vi "FDD Self TRAINING Parse Datafile Into BINS Ver05.vi"(9 "Zone Density \n(KEEP Closest # Points)":i32=5, 10 "Data BINS Defined - ARRAY":T2(array[cluster])=[{"Datafile COL"=182.0, "Start Center Value"=60.0, "Bin Width"=5.0, "End Center Value"=100.0}, {"Datafile COL"=83.0, "Start Center Value"=40.0, "Bin Width"=5.0, "End Center Value"=100.0}, {"Datafile COL"=195.0, "Start Center Value"=60.0, "Bin Width"=5.0, "End Center Value"=120.0}], 11 "Input Datafile":path=path "C:/Vance/FDD Split System Project/FDD_LOW-HIGH_EfficiencyHP_Testing/Goodman 14SEER/SHORT LINESET DATA/COOLING/NF - No Fault Cooling Test DATA/NF-SHORT-COOL-SSData 170719a.txt") -> (3 "BEST (Closest in Datafile) Array - String with BIN ASSIGNMENTS":string[][](array[string]), 4 "Each BIN Best Points Array - STRING":string[][](array[string]), 5 "ALL BINS as DEFINED by Start, Width and End, Array - Numeric":dbl[][](array[numeric]))   [LabVIEW 2017]
uses:
  <vilib>/Analysis/Matrix/Datatypes/RealMatrix.ctl
  <vilib>/Utility/file.llb/Read Delimited Spreadsheet (string).vi
  <vilib>/Analysis/Matrix/Numeric/Conversions/Array To Matrix - RA.vi
  <vilib>/Analysis/Matrix/Numeric/Conversions/Matrix To Array - RM.vi
  <vilib>/Utility/file.llb/Write Delimited Spreadsheet (string).vi
  <vilib>/Analysis/Matrix/NI_Matrix.lvlib
  <vilib>/Analysis/NI_AALBase.lvlib
panel:
  out "Total # POINTS":i32
  out "Total # of BINS":i32
  out "Total # POINTS\nKEPT out of\nCurrent Datafile":i32
  out "# RAW Data ROWS":i32
  out "Dmax":dbl format="%.3f"
  out "% Retained":dbl format="%#.2f"
  out "TIME to PARSE (sec)":dbl format="%.2f"
  out "Processing":string
  out "Current Datafile":string
  out "Running":bool
  in  "Tab Control":T1(tab)
  in  "Delete Bins Where\nIndependent Variable #1 > #0":bool=TRUE
  out "Datafile Array - String":string[][](array[string])
  in  "Delete Bins Where\nIndependent Variable #2 > #1":bool
  in  "Delete Bins Where\nIndependent Variable #2 < #0":bool=TRUE
  out "Each Point in Just ONE BIN\n(Distance, BIN#, POINT#)":dbl[][](array[numeric])
  out "BIN RANGES as DEFINED by Start, Width and End Array - Numeric":dbl[][](array[numeric])
  out "RAW Data COLS Selected to be Put into BINS Array - String":string[][](array[string])
  out "Raw Independent Variables STATISTICS - Array":T3(array[cluster])
  out "EACH BIN \nHas X Best\nPOINTS":i32
  out "ALL BINS (Distance, BIN#, POINT#)":dbl[][](array[numeric])
  out "FILTERED by DMAX with Same Point in Multiple BINS Possibly\nDISTANCE, BIN#, POINT# (DATA ARRAY INDEX)":dbl[][](array[numeric])
  out "RAW Data COLS Selected to be Put into BINS Array - String 2":string[][](array[string])
  out "BINNED Data STATISTICS - Array":T3(array[cluster])
  out "PDF Filename":string
  in  "Create PDF Report":bool
  in  "SAVE File":bool
  in  "SAVED Data BINS File Path Control":path
  out "SAVE FILE error out":errorcluster
  out "CREATE JPG error out":errorcluster
  # "Define the BINS.  BIN has a Start Center Value, End Center Value, and Bin Width."
  # "This allows me to delete BINS where\nthe indoor dewpoint is greater than the dry-bulb, or \nwhere outdoor dry-bulb is less than indoor dry-bulb."
  # "POINT# corresponds to this ROW#-1"
  # "NOT BIN CENTER Coordinate\n(99.99 Indicates EMPTY CELL)"
  # "BIN#"
  # "POINT# corresponds to this ROW#-1"
  # "DISTANCE"
  # "Point# Correspondes to the INDEX of \nthe ARRAY to the RIGHT (not including \nheader label, INDEX 0 is row 2)"
  # "Distance from BIN Center to ANY Point\nD = sqrt((b1-p1)^2 + (b2-p2)^2 + (b3-p3)^2 + .......)\nwhere b# is BIN coordinate and p# is point coordinate in \nthe multi-dimensional space."
  # "Maximum D (distance) is defined by the BIN WIDTHS:\nfor example in a 3D space (x,y,z) with BIN WIDTHS of\n(dx = 5, dy = 5, dz = 5), the MAX D would equal, \nDmax = sqrt (5^2 + 5^2 + 5^2)/2 = sqrt (75)/2 = 4.33.\nIn order to keep the n best points, the distance satisfies the following:\n       0<= D < Dmax"
  # "Calculate Distance of Each Point to \nthe Center of the BIN and Keep the\nBEST Points"
  # "Error is okay here.\nJust means JPEG \nDIRECTORY HAD to \nbe created."
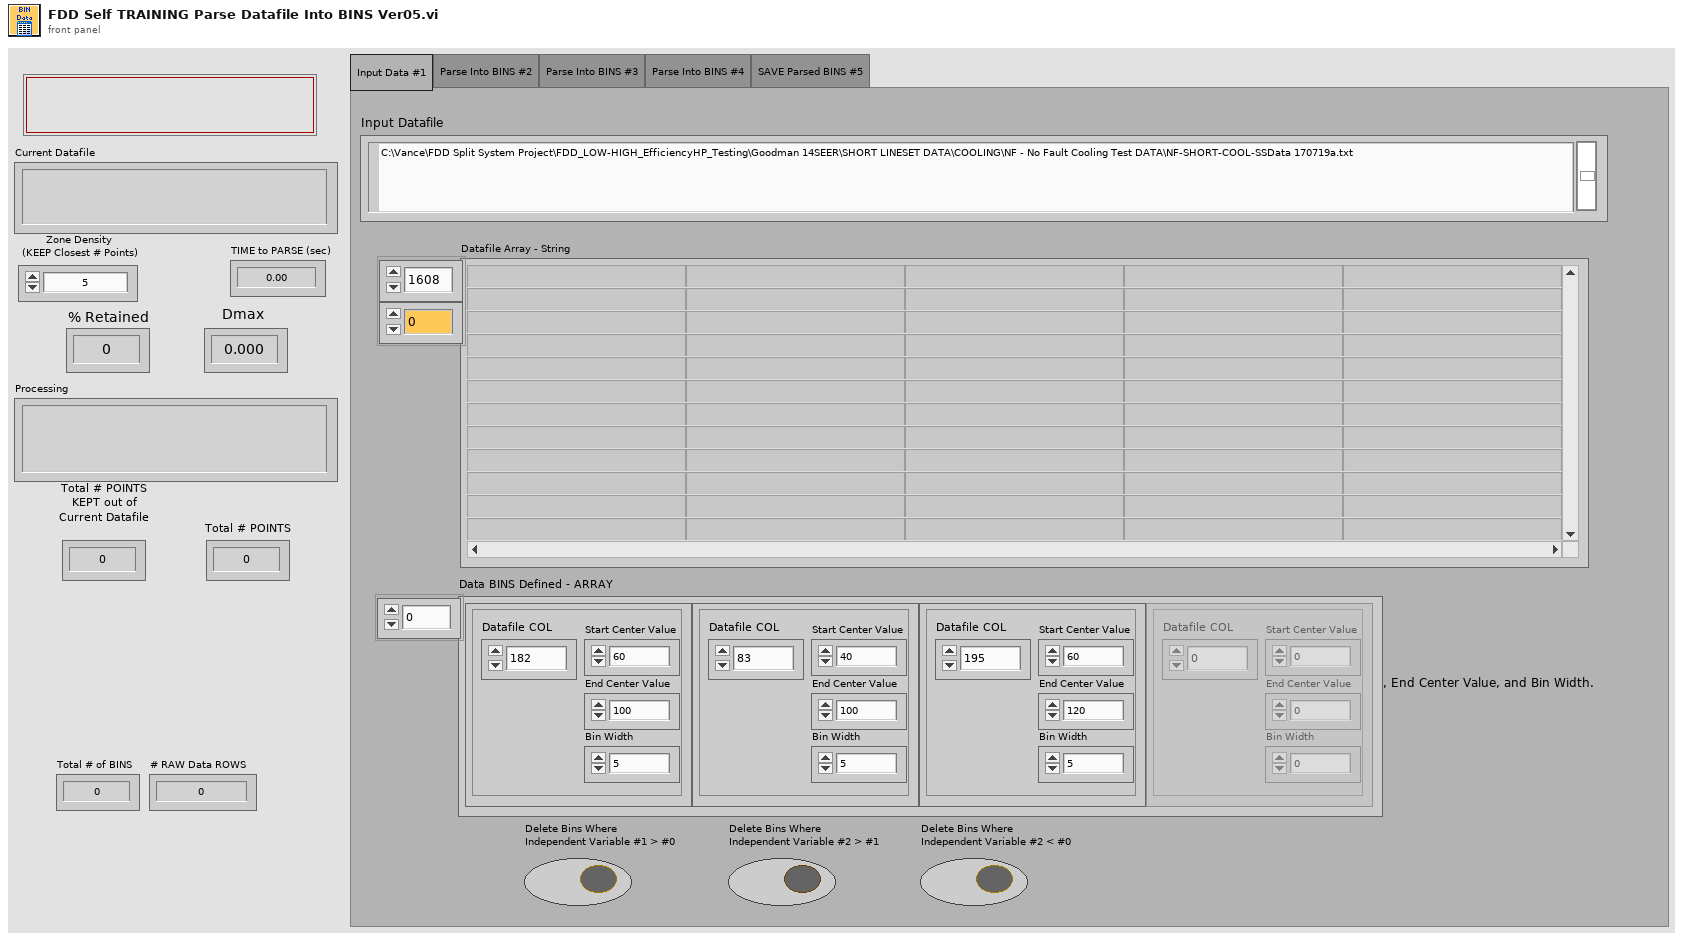
[diagram p1: front panel]
types:
  T1 = enum32{"Input Data #1", "Parse Into BINS #2", "Parse Into BINS #3", "Parse Into BINS #4", "SAVE Parsed BINS #5"}
  T2 = cluster{"Datafile COL":dbl, "Start Center Value":dbl, "Bin Width":dbl, "End Center Value":dbl}[]
  T3 = cluster{"Header":string, "Mean":dbl, "Std. Dev":dbl, "MAX":dbl, "MIN":dbl, "Range":dbl}[]
  T4 = typedef "NI_Matrix.lvlib/RealMatrix.ctl" = dbl[][]
  T5 = cluster{"String":string, "mean":dbl, "standard deviation":dbl, dbl, dbl, dbl}
  T6 = typedef "imagedata.ctl" = cluster{"image type":i32, "image depth":i32, "image":u8[], "mask":u8[], "colors":u32[], "Rectangle":cluster{"left":i16, "top":i16, "right":i16, "bottom":i16}}
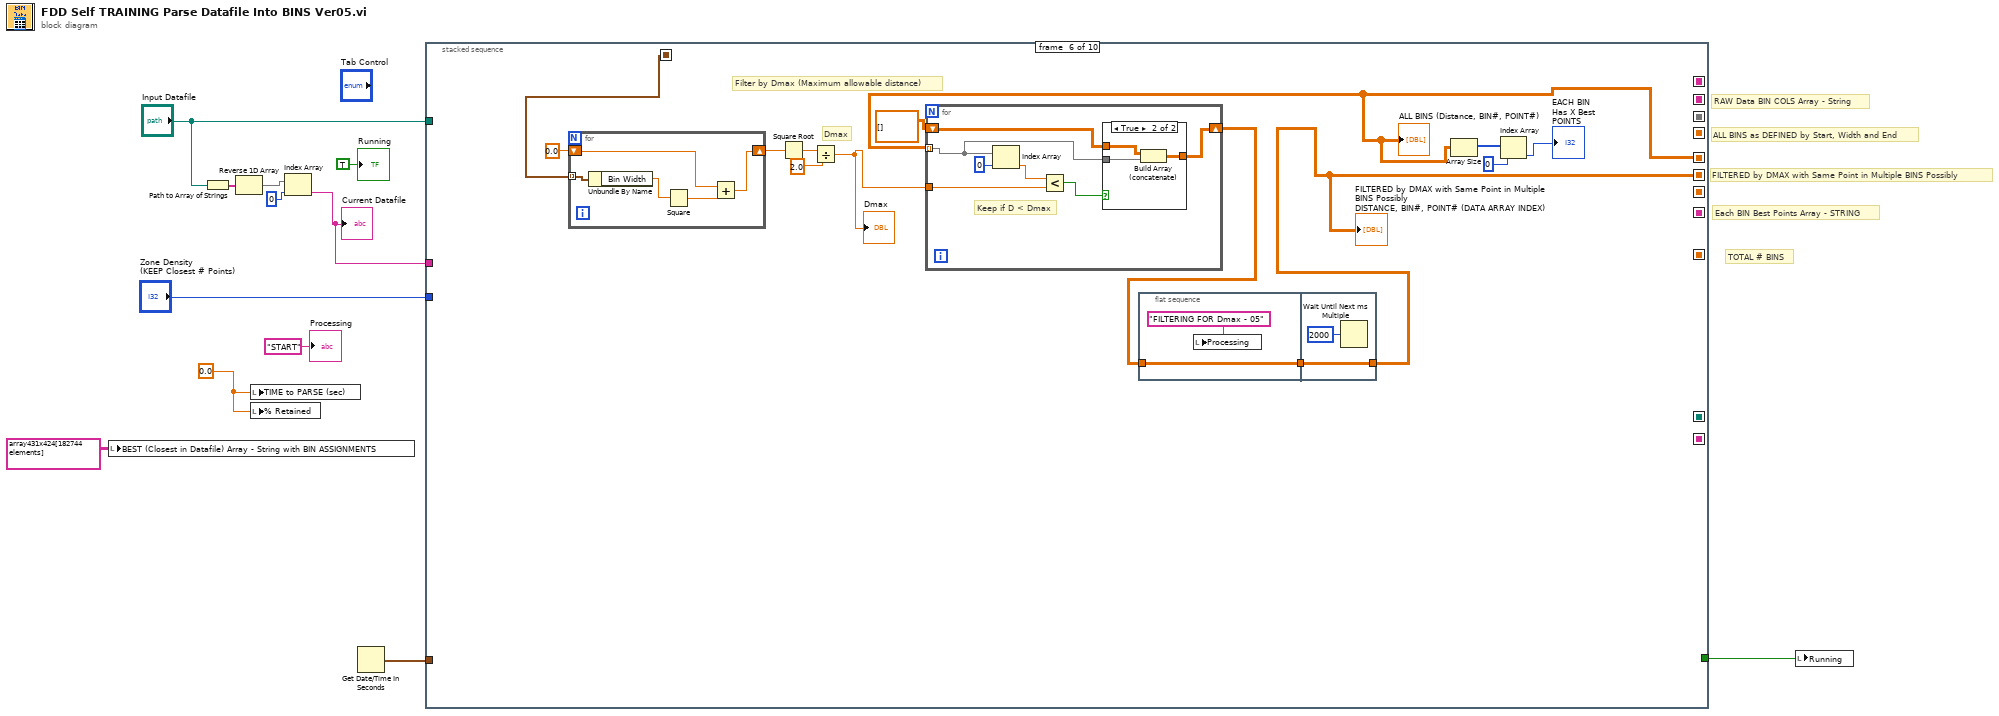
[diagram p0: block diagram]
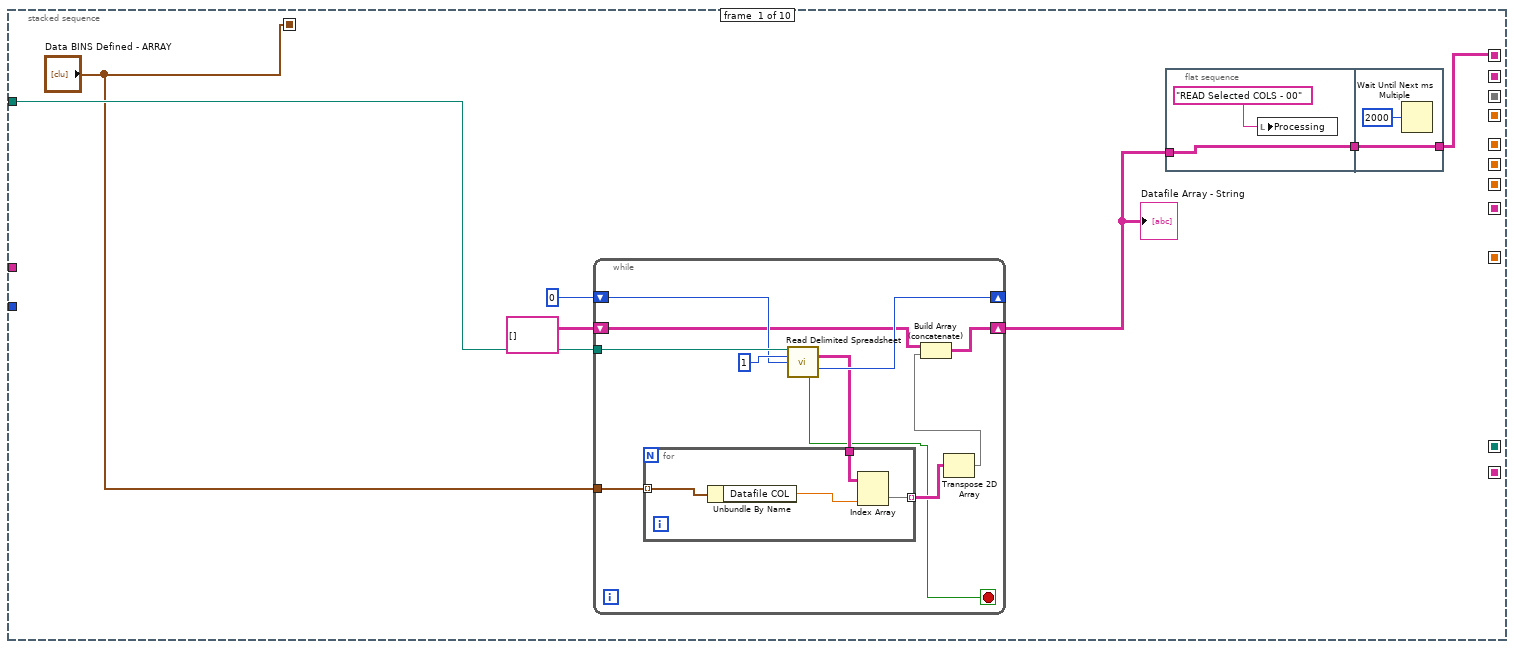
[diagram p2: hidden frame]
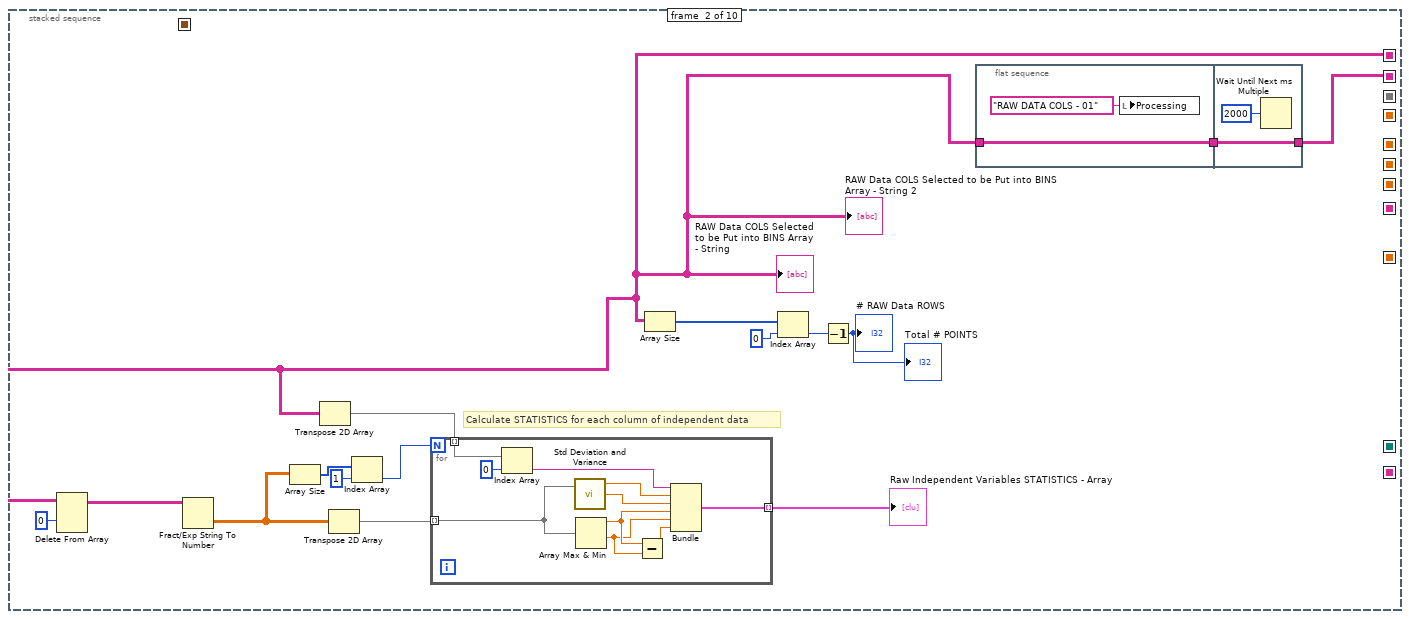
[diagram p3: hidden frame]
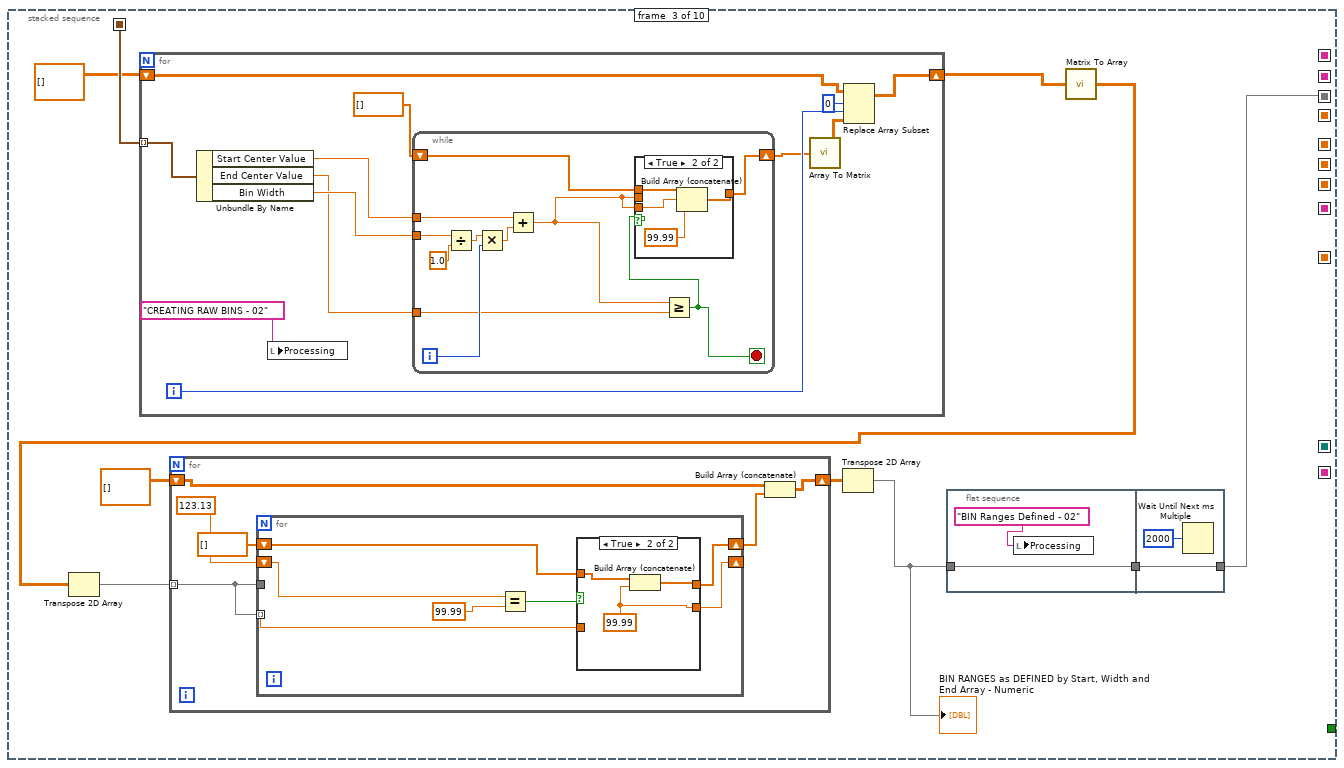
[diagram p4: hidden frame]
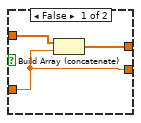
[diagram p5: hidden frame]
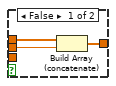
[diagram p6: hidden frame]
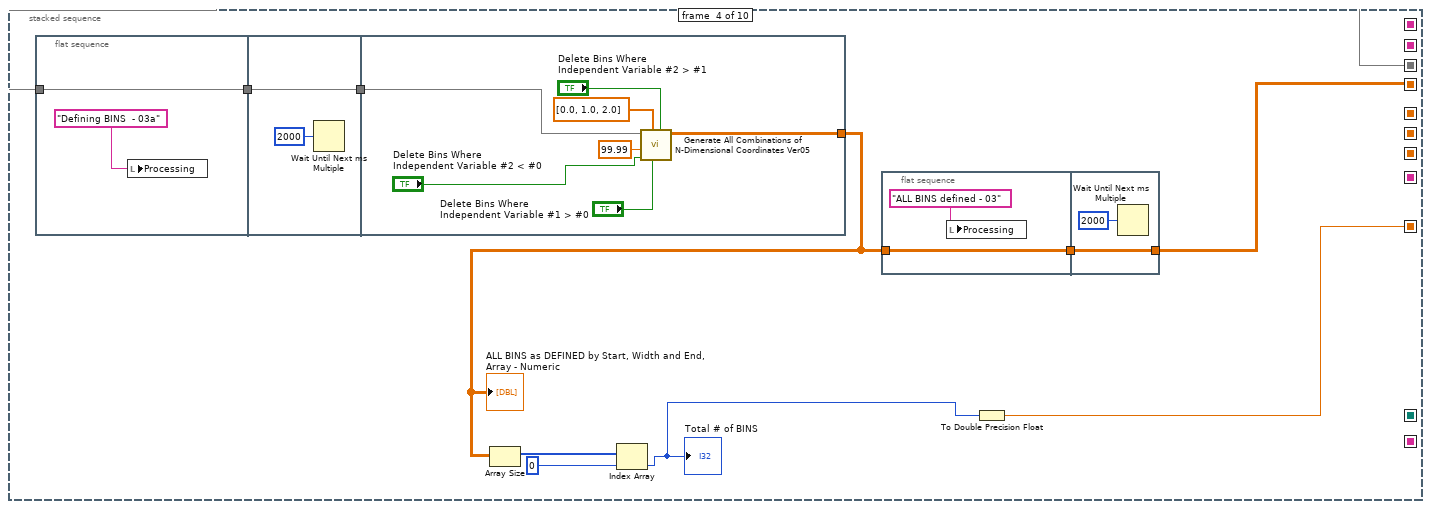
[diagram p7: hidden frame]
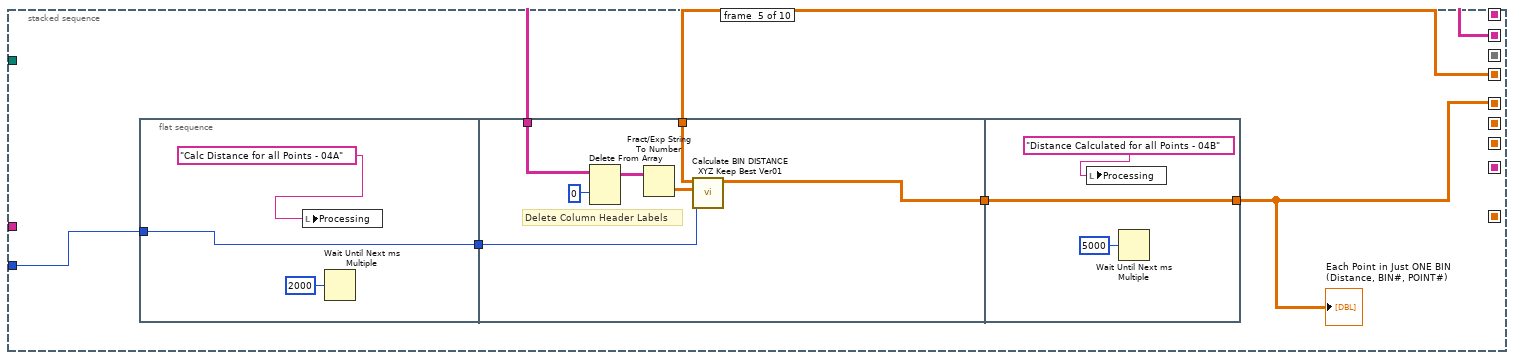
[diagram p8: hidden frame]
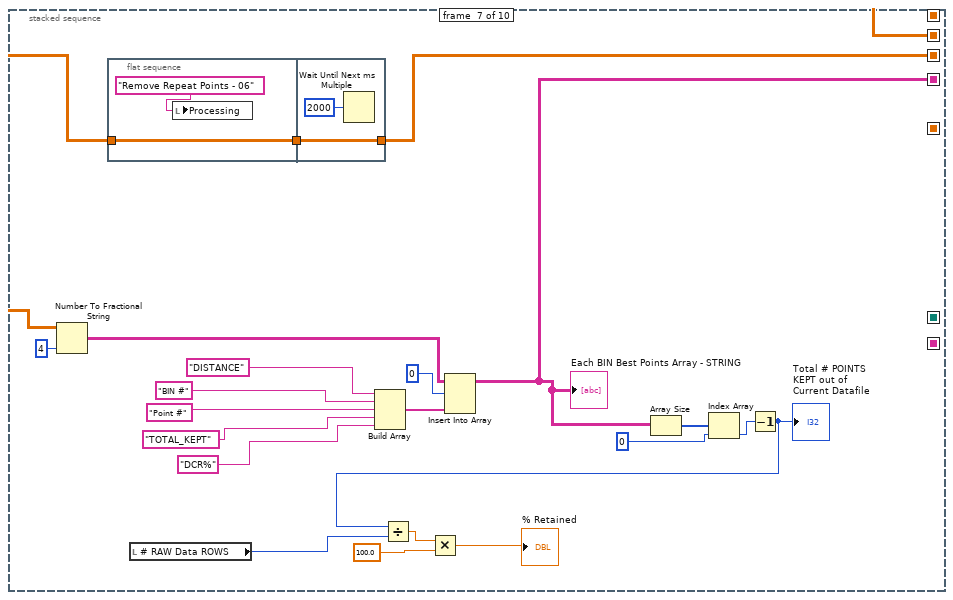
[diagram p10: hidden frame]
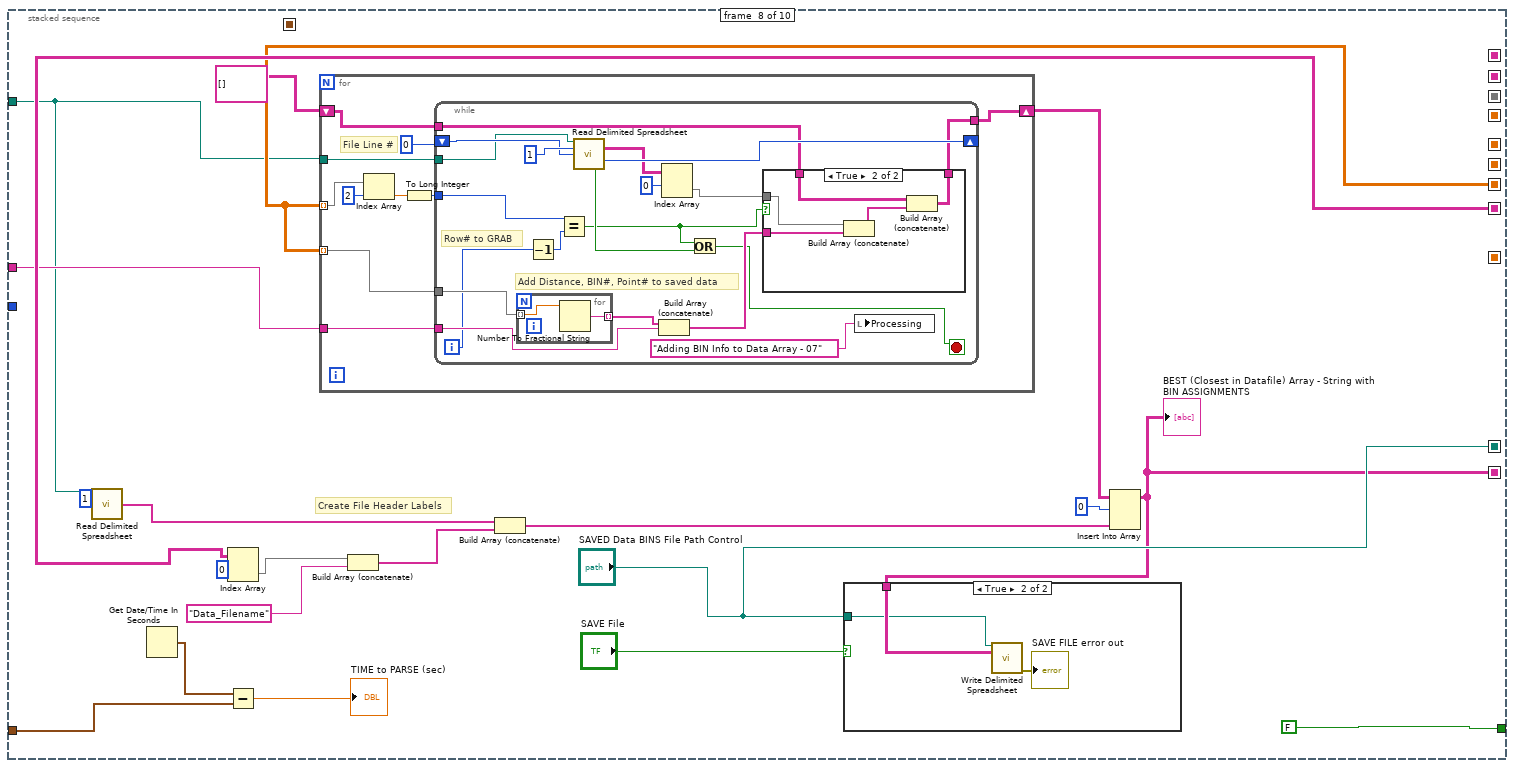
[diagram p11: hidden frame]
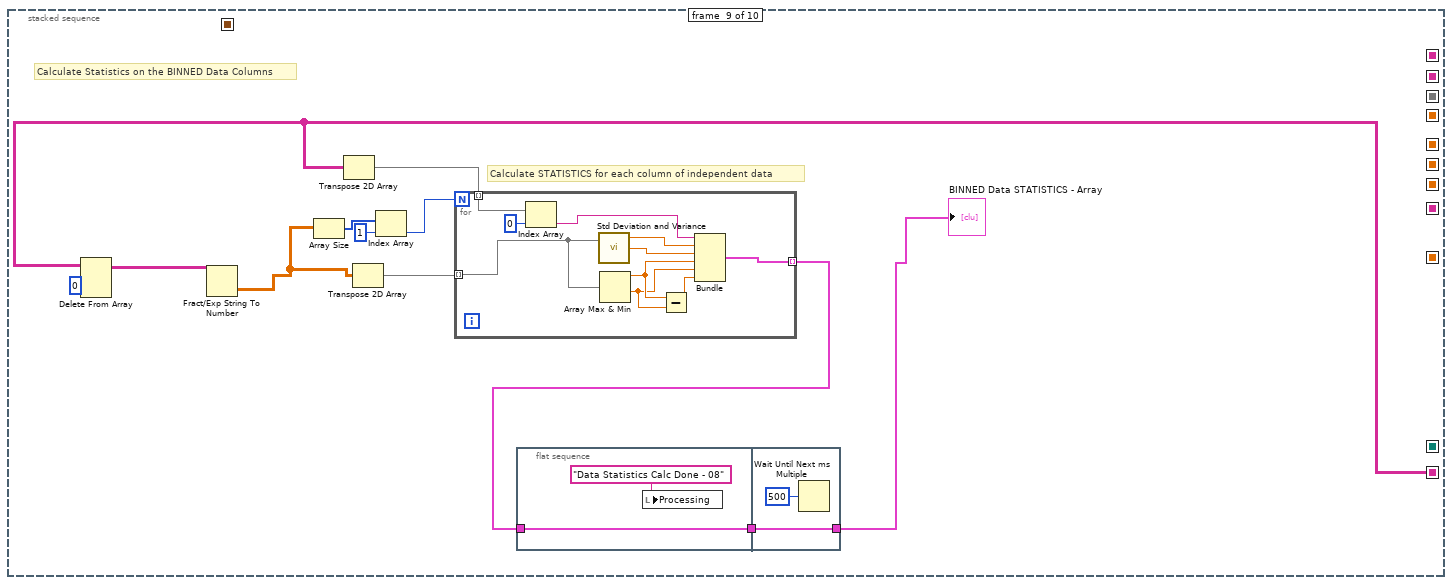
[diagram p14: hidden frame]
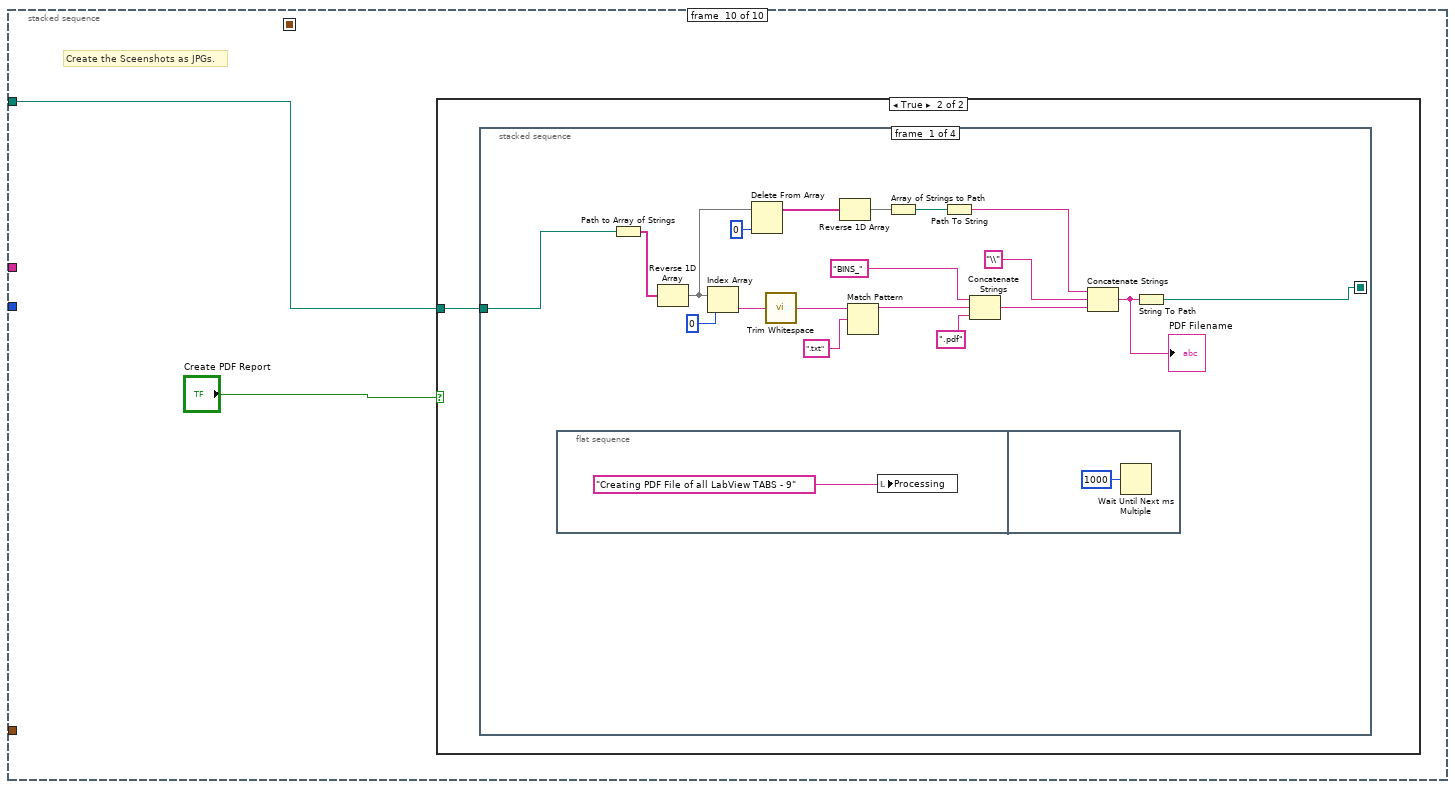
[diagram p15: hidden frame]
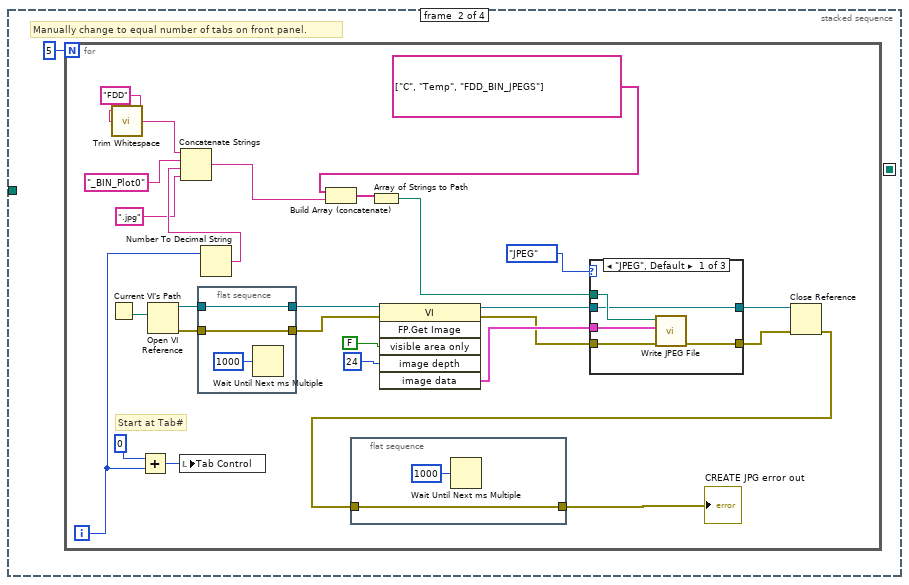
[diagram p17: hidden frame]
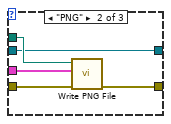
[diagram p18: hidden frame]
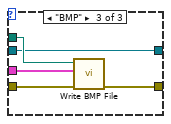
[diagram p19: hidden frame]
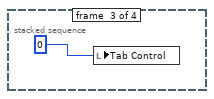
[diagram p20: hidden frame]
diagram:
  w2 = 0.0 ("TIME to PARSE (sec)")
  # "TOTAL # BINS"
  # "Each BIN Best Points Array - STRING"
  # "FILTERED by DMAX with Same Point in Multiple BINS Possibly"
  # "ALL BINS as DEFINED by Start, Width and End"
  # "RAW Data BIN COLS Array - String"
  n1 = local write "BEST (Closest in Datafile) Array - String with BIN ASSIGNMENTS"(string[][] array431x424[182744 elements] ("BEST (Closest in Datafile) Array - String with BIN ASSIGNMENTS")) -> ()
  n2 = Path to Array of Strings(0:"Input Datafile") -> (2:w9:string[])  [unwired: 1 out]
  n3 = Reverse 1D Array(array=w9) -> (reversed array=w8:string[])
  n4 = local write "TIME to PARSE (sec)"(w2) -> ()
  n5 = local write "% Retained"(w2) -> ()
  n6 = Index Array(array=w8, index=0) -> (element=w3:string)
  "Current Datafile" <- w3
  n7 = Get Date/Time In Seconds() -> (seconds since 1Jan1904=w5:timestamp)
  n8 = stacked-sequence {
    seq-local: [w13 _ _ _ _ _ _ _ _ _] -> [_ w41 _ _ _ _ _ _ _ _]
    seq-local: [_ w40 _ _ _ _ _ _ _ _] -> [_ _ _ _ w161 _ _ _ _ _]
    seq-local: ["Data BINS Defined - ARRAY" _ _ _ _ _ _ _ _ _] -> [_ _ w78 _ _ w189 _ _ _ _]
    seq-local: [_ _ w71 _ _ _ _ _ _ _] -> [_ _ _ w135 _ _ _ _ _ _]
    seq-local: [_ _ _ w138 _ _ _ _ _ _] -> [_ _ _ _ w160 _ _ _ _ _]
    seq-local: [_ _ _ _ w157 _ _ _ _ _] -> [_ _ _ _ _ w180 _ _ _ _]
    seq-local: [_ _ _ _ _ w176 _ _ _ _] -> [_ _ _ _ _ _ w210 _ _ _]
    seq-local: [_ _ _ _ _ _ w213 _ _ _] -> [_ _ _ _ _ _ _ w240 _ _]
    seq-local: [_ _ _ _ _ _ w220 _ _ _] -> [_ _ _ _ _ _ _ w248 _ _]
    seq-local: [_ _ _ _ _ _ _ "SAVED Data BINS File Path Control" _ _] -> [_ _ _ _ _ _ _ _ _ _]
    seq-local: [_ _ _ _ _ _ _ w241 _ _] -> [_ _ _ _ _ _ _ _ w300 _]
    seq-local: [_ _ _ w132 _ _ _ _ _ _] -> [_ _ _ _ _ _ _ _ _ _]
    tunnel: "Input Datafile" -> [w19 _ _ _ _ _ _ w237 _ w323]
    tunnel: [_ _ _ _ _ _ _ FALSE ("Running") _ _] -> w12
    tunnel: "Zone Density \n(KEEP Closest # Points)" -> [_ _ _ _ w159 _ _ _ _ _]
    tunnel: w5 -> [_ _ _ _ _ _ _ w252 _ _]
    tunnel: w3 -> [_ _ _ _ _ _ _ w247 _ _]
    frame #0 {
      n9 = while {
        tunnel: w19 -> [w34]
        shift-right: [w32] -> _
        shift-left: 0 ("mark after read (chars.)") -> [w31]
        shift-right: [w30] -> w14
        shift-left: string[][] [] -> [w29]
        tunnel: "Data BINS Defined - ARRAY" -> [w27]
        stop <- w24 stop-if-true
        n10 = call-poly <vilib>:"Read Delimited Spreadsheet.vi"("file path (dialog if empty)"=w34, "number of rows (all:-1)"=1, "start of read offset (chars.:0)"=w31) -> ("all rows"=w28:string[][], "mark after read (chars.)"=w32:i32, "EOF?"=w24:bool)  [unwired: 7 in, 3 out]
        n11 = for {
          tunnel: w27 -> [w38] mode=indexing
          tunnel: w28 -> [w37]
          tunnel: [w36] -> w26 mode=indexing
          n12 = Unbundle By Name(w38) -> ("Datafile COL"=w35:dbl)
          n13 = Index Array(array=w37, index (col)=w35) -> (element=w36:string[])  [unwired: 1 in]
        }
        n14 = Transpose 2D Array(2D array=w26) -> (transposed array=w25:string[][])
        n15 = Build Array (concatenate)(w29, w25) -> (w30:string[][])
      }
      "Datafile Array - String" <- w14
      n16 = flat-sequence {
        tunnel: [w21] -> w15
        tunnel: w14 -> [w21]
        tunnel: [w22] -> w13
        tunnel: w15 -> [w22]
        frame #0 {
          n17 = local write "Processing"("READ Selected COLS - 00") -> ()
        }
        frame #1 {
          n18 = Wait Until Next ms Multiple(millisecond multiple=u32 2000) -> ()  [unwired: 1 out]
        }
      }
    }
    frame #1 {
      # "Calculate STATISTICS for each column of independent data"
      n19 = Delete From Array "Delete From Array"(array=w41, index (row)=0) -> (array with subset deleted=w50:string[][])  [unwired: 2 in, 1 out]
      n20 = Fract/Exp String To Number(string=w50) -> (number=w46:dbl[][])  [unwired: 3 in, 1 out]
      n21 = Array Size(array=w46) -> (size(s)=w49:i32[])
      n22 = Transpose 2D Array(2D array=w41) -> (transposed array=w44:string[][])
      n23 = Transpose 2D Array(2D array=w46) -> (transposed array=w45:dbl[][])
      n24 = Index Array(array=w49, index=1) -> (element=w47:i32)
      n25 = for {
        N: w47 -> [_]
        tunnel: w45 -> [w66] mode=indexing
        tunnel: [w62] -> w43 mode=indexing
        tunnel: w44 -> [w61] mode=indexing
        n26 = Index Array(array=w61, index=0) -> (element=w59:string)
        n27 = call <vilib>:"Std Deviation and Variance.vi"("X"=w66) -> ("mean"=w68:dbl, "standard deviation"=w67:dbl)  [unwired: 1 in, 1 out]
        n28 = Array Max & Min(array=w66) -> (max value=w65:dbl, min value=w64:dbl)  [unwired: 2 out]
        n29 = Subtract(x=w65, y=w64) -> (x-y=w63:dbl)
        n30 = Bundle("String"=w59, "mean"=w68, "standard deviation"=w67, w65, w64, w63) -> (w62:T5)  [unwired: 1 in]
      }
      "Raw Independent Variables STATISTICS - Array" <- w43
      n31 = Array Size(array=w41) -> (size(s)=w54:i32[])
      n32 = Index Array(array=w54, index=0) -> (element=w52:i32)
      n33 = Decrement(x=w52) -> (x-1=→"# RAW Data ROWS" →"Total # POINTS":i32)
      n34 = flat-sequence {
        tunnel: [w56] -> w42
        tunnel: w41 -> [w56]
        tunnel: [w57] -> w40
        tunnel: w42 -> [w57]
        frame #0 {
          n35 = local write "Processing"("RAW DATA COLS - 01" ("Processing")) -> ()
        }
        frame #1 {
          n36 = Wait Until Next ms Multiple(millisecond multiple=u32 2000) -> ()  [unwired: 1 out]
        }
      }
      "RAW Data COLS Selected to be Put into BINS Array - String" <- w41
      "RAW Data COLS Selected to be Put into BINS Array - String 2" <- w41
    }
    frame #2 {
      n37 = for {
        tunnel: w78 -> [w113] mode=indexing
        shift-right: [w105] -> w76
        shift-left: T4 [] ("Real Matrix") -> [w104]
        i -> [w108]
        n38 = Unbundle By Name(w113) -> ("Start Center Value"=w112:dbl, "End Center Value"=w109:dbl, "Bin Width"=w111:dbl)
        n39 = local write "Processing"("CREATING RAW BINS - 02" ("Processing")) -> ()
        n40 = while {
          shift-right: [w121] -> w107
          shift-left: dbl[] [] -> [w120]
          tunnel: w112 -> [w124]
          tunnel: w111 -> [w116]
          tunnel: w109 -> [w119]
          i -> [w122]
          stop <- w118 stop-if-true
          n41 = Divide(x=w116, y=1.0) -> (x/y=w114:dbl)
          n42 = Multiply(x=w114, y=w122) -> (x*y=w123:dbl)
          n43 = Add(x=w124, y=w123) -> (x+y=w117:dbl)
          n44 = Greater Or Equal?(x=w117, y=w119) -> (x >= y?=w118:bool)
          n45 = case shown="True" w118 {
            tunnel: [w127 w130] -> w121
            tunnel: w120 -> [w126 w131]
            tunnel: w117 -> [w125 _]
            tunnel: w117 -> [_ w129]
            frame False {
              n46 = Build Array (concatenate)(w126, w125) -> (w127:dbl[])
            }
            frame True {
              n47 = Build Array (concatenate)(w131, w129, 99.99 ("element")) -> (w130:dbl[])
            }
          }
        }
        n48 = call-poly <vilib>:"Array To Matrix.vi"("Real 1D Array"=w107) -> ("Real Matrix (Column Vector)"=w106:T4)
        n49 = Replace Array Subset(array=w104, new element=w106, index (row)=0 ("disabled index (row)"), index (col)=w108) -> (w105:T4)
      }
      n50 = flat-sequence {
        tunnel: [w80] -> w70
        tunnel: w69 -> [w80]
        tunnel: [w81] -> w71
        tunnel: w70 -> [w81]
        frame #0 {
          n51 = local write "Processing"("BIN Ranges Defined - 02") -> ()
        }
        frame #1 {
          n52 = Wait Until Next ms Multiple(millisecond multiple=u32 2000) -> ()  [unwired: 1 out]
        }
      }
      n53 = call-poly <vilib>:"Matrix To Array.vi"("Real Matrix"=w76) -> ("Real 2D Array"=w72:dbl[][])
      n54 = Transpose 2D Array(2D array=w72) -> (transposed array=w75:dbl[][])
      n55 = for {
        tunnel: w75 -> [w88] mode=indexing
        shift-right: [w86] -> w73
        shift-left: dbl[][] [] -> [w84]
        n56 = for {
          tunnel: w88 -> [_]
          tunnel: w88 -> [w94] mode=indexing
          shift-right: [w92] -> w85
          shift-left: dbl[] [] -> [w91]
          shift-right: [w90] -> _
          shift-left: 123.13 -> [w95]
          n57 = Equal?(x=w95, y=99.99) -> (x = y?=w93:bool)
          n58 = case shown="True" w93 {
            tunnel: w94 -> [w96 _]
            tunnel: [w98 w100] -> w92
            tunnel: w91 -> [w97 w101]
            tunnel: [w96 w99] -> w90
            frame False {
              n59 = Build Array (concatenate)(w97, w96) -> (w98:dbl[])
            }
            frame True {
              w99 = 99.99 ("y")
              n60 = Build Array (concatenate)(w101, w99) -> (w100:dbl[])
            }
          }
        }
        n61 = Build Array (concatenate)(w84, w85) -> (w86:dbl[][])
      }
      n62 = Transpose 2D Array(2D array=w73) -> (transposed array=w69:dbl[][])
      "BIN RANGES as DEFINED by Start, Width and End Array - Numeric" <- w69
    }
    frame #3 {
      n63 = flat-sequence {
        tunnel: [w143] -> w137
        tunnel: w135 -> [w143]
        tunnel: w137 -> [w145]
        tunnel: [w145] -> w136
        tunnel: w136 -> [w148]
        tunnel: [w147] -> w134
        frame #0 {
          n64 = local write "Processing"("Defining BINS  - 03a") -> ()
        }
        frame #1 {
          n65 = Wait Until Next ms Multiple(millisecond multiple=u32 2000) -> ()  [unwired: 1 out]
        }
        frame #2 {
          n66 = call "Generate All Combinations of N-Dimensional Coordinates Ver05.vi"("Delete ROWS w/\nCOL #2 > #1"="Delete Bins Where\nIndependent Variable #2 > #1", "Delete ROWS w/\nCOL #1 > #0"="Delete Bins Where\nIndependent Variable #1 > #0", "INDEX of \nCOLS to Use"=dbl[] [0.0, 1.0, 2.0] ("INDEX of \nCOLS to Use"), "Delete ROWS w/\nCOL #2 < #0"="Delete Bins Where\nIndependent Variable #2 < #0", "Delete ROW if\nContains #"=99.99 ("Delete ROW if\nContains #"), "2D Big Data Array"=w148) -> ("FINAL ARRAY"=w147:dbl[][])  [unwired: 4 in]
        }
      }
      n67 = Array Size(array=w134) -> (size(s)=w141:i32[])
      n68 = Index Array(array=w141, index=0) -> (element=w133:i32)
      "Total # of BINS" <- w133
      n69 = flat-sequence {
        tunnel: [w154] -> w139
        tunnel: w134 -> [w154]
        tunnel: [w155] -> w138
        tunnel: w139 -> [w155]
        frame #0 {
          n70 = local write "Processing"("ALL BINS defined - 03") -> ()
        }
        frame #1 {
          n71 = Wait Until Next ms Multiple(millisecond multiple=u32 2000) -> ()  [unwired: 1 out]
        }
      }
      n72 = To Double Precision Float(number=w133) -> (double precision float=w132:dbl)
      "ALL BINS as DEFINED by Start, Width and End, Array - Numeric" <- w134
    }
    frame #4 {
      n73 = flat-sequence {
        tunnel: w159 -> [w164]
        tunnel: [w164] -> w158
        tunnel: [w166] -> w162
        tunnel: w161 -> [w169]
        tunnel: w160 -> [w168]
        tunnel: w158 -> [w167]
        tunnel: w162 -> [w175]
        tunnel: [w175] -> w157
        frame #0 {
          n74 = local write "Processing"("Calc Distance for all Points - 04A") -> ()
          n75 = Wait Until Next ms Multiple(millisecond multiple=u32 2000) -> ()  [unwired: 1 out]
        }
        frame #1 {
          # "Delete Column Header Labels"
          n76 = Delete From Array(array=w169, index (row)=0) -> (array with subset deleted=w171:string[][])  [unwired: 2 in, 1 out]
          n77 = Fract/Exp String To Number(string=w171) -> (number=w172:dbl[][])  [unwired: 3 in, 1 out]
          n78 = call "Calculate BIN DISTANCE XYZ Keep Best Ver01.vi"("KEEP X Best Points\nfor EACH BIN"=w167, "Data (X,Y,Z)"=w172, "BIN (X,Y,Z)"=w168) -> ("Duplicate Points ELIMINATED"=w166:dbl[][])  [unwired: 8 in]
        }
        frame #2 {
          n79 = local write "Processing"("Distance Calculated for all Points - 04B") -> ()
          n80 = Wait Until Next ms Multiple(millisecond multiple=u32 5000) -> ()  [unwired: 1 out]
        }
      }
      "Each Point in Just ONE BIN\n(Distance, BIN#, POINT#)" <- w157
    }
    frame #5 {
      # "Dmax"
      # "Filter by Dmax (Maximum allowable distance)"
      n81 = for {
        tunnel: w189 -> [w209] mode=indexing
        shift-right: [w206] -> w187
        shift-left: 0.0 -> [w205]
        n82 = Unbundle By Name(w209) -> ("Bin Width"=w207:dbl)
        n83 = Square(x=w207) -> (x^2=w208:dbl)
        n84 = Add(x=w205, y=w208) -> (x+y=w206:dbl)
      }
      n85 = Square Root(x=w187) -> (sqrt(x)=w185:dbl)
      n86 = Divide(x=w185, y=2.0) -> (x/y=w183:dbl)
      "Dmax" <- w183
      n87 = for {
        tunnel: w180 -> [w196] mode=indexing
        shift-right: [w195] -> w177
        shift-left: dbl[][] [] -> [w194]
        tunnel: w183 -> [w198]
        # "Keep if D < Dmax"
        n88 = Index Array(array=w196, index=0) -> (element=w199:dbl)
        n89 = Less?(x=w199, y=w198) -> (x < y?=w197:bool)
        n90 = case shown="True" w197 {
          tunnel: w196 -> [_ w204]
          tunnel: [w201 w203] -> w195
          tunnel: w194 -> [w201 w202]
          frame False {
          }
          frame True {
            n91 = Build Array (concatenate)(w202, w204) -> (w203:dbl[][])
          }
        }
      }
      n92 = flat-sequence {
        tunnel: [w191] -> w178
        tunnel: w177 -> [w191]
        tunnel: [w192] -> w176
        tunnel: w178 -> [w192]
        frame #0 {
          n93 = local write "Processing"("FILTERING FOR Dmax - 05" ("Processing")) -> ()
        }
        frame #1 {
          n94 = Wait Until Next ms Multiple(millisecond multiple=u32 2000) -> ()  [unwired: 1 out]
        }
      }
      n95 = Array Size(array=w180) -> (size(s)=w182:i32[])
      n96 = Index Array(array=w182, index=0) -> (element=→"EACH BIN \nHas X Best\nPOINTS":i32)
      "FILTERED by DMAX with Same Point in Multiple BINS Possibly\nDISTANCE, BIN#, POINT# (DATA ARRAY INDEX)" <- w176
      "ALL BINS (Distance, BIN#, POINT#)" <- w180
    }
    frame #6 {
      n97 = Number To Fractional String(number=w210, precision (6)=i16 4) -> (F-format string=w223:string[][])  [unwired: 2 in]
      n98 = flat-sequence {
        tunnel: [w231] -> w214
        tunnel: w210 -> [w231]
        tunnel: [w233] -> w213
        tunnel: w214 -> [w233]
        frame #0 {
          n99 = local write "Processing"("Remove Repeat Points - 06") -> ()
        }
        frame #1 {
          n100 = Wait Until Next ms Multiple(millisecond multiple=u32 2000) -> ()  [unwired: 1 out]
        }
      }
      n101 = local read "# RAW Data ROWS"() -> (w218:i32)
      n102 = Build Array("DISTANCE", "BIN #", "Point #", "TOTAL_KEPT", "DCR%") -> (w225:string[])
      n103 = Insert Into Array "Insert Into Array"(array=w223, index (row)=0, new element=w225) -> (w220:string[][])  [unwired: 1 in]
      "Each BIN Best Points Array - STRING" <- w220
      n104 = Array Size(array=w220) -> (size(s)=w222:i32[])
      n105 = Index Array(array=w222, index=0) -> (element=w221:i32)
      n106 = Decrement(x=w221) -> (x-1=w219:i32)
      "Total # POINTS\nKEPT out of\nCurrent Datafile" <- w219
      n107 = Divide(x=w219, y=w218) -> (x/y=w217:dbl)
      n108 = Multiply(x=w217, y=100.0) -> (x*y=→"% Retained":dbl)
    }
    frame #7 {
      # "Create File Header Labels"
      n109 = call-poly <vilib>:"Read Delimited Spreadsheet.vi"("file path (dialog if empty)"=w237, "number of rows (all:-1)"=1) -> ("first row"=w236:string[])  [unwired: 8 in, 5 out]
      n110 = Get Date/Time In Seconds() -> (seconds since 1Jan1904=w254:timestamp)
      n111 = Index Array(array=w248, index (row)=0) -> (element=w245:string[])  [unwired: 1 in]
      n112 = Subtract(x=w254, y=w252) -> (x-y=→"TIME to PARSE (sec)":dbl)
      n113 = for {
        tunnel: w240 -> [w260] mode=indexing
        tunnel: w247 -> [w265]
        tunnel: w237 -> [w263]
        tunnel: w240 -> [w259] mode=indexing
        shift-right: [w257] -> w238
        shift-left: string[][] [] -> [w256]
        # "File Line #"
        n114 = Index Array(array=w260, index=2) -> (element=w262:dbl)
        n115 = To Long Integer(number=w262) -> (32bit integer=w258:i32)
        n116 = while {
          tunnel: w259 -> [w285]
          tunnel: w265 -> [w283]
          shift-right: [w279] -> _
          shift-left: 0 ("number of rows (all:-1)") -> [w280]
          tunnel: w263 -> [w276]
          tunnel: w258 -> [w275]
          tunnel: [w271] -> w257
          tunnel: w256 -> [w270]
          i -> [w278]
          stop <- w272 stop-if-true
          # "Add Distance, BIN#, Point# to saved data"
          # "Row# to GRAB"
          n117 = for {
            tunnel: w285 -> [w293] mode=indexing
            tunnel: [w292] -> w284 mode=indexing
            n118 = Number To Fractional String(number=w293) -> (F-format string=w292:string)  [unwired: 3 in]
          }
          n119 = Decrement(x=w278) -> (x-1=w277:i32)
          n120 = Equal?(x=w275, y=w277) -> (x = y?=w273:bool)
          n121 = call-poly <vilib>:"Read Delimited Spreadsheet.vi"("file path (dialog if empty)"=w276, "number of rows (all:-1)"=1, "start of read offset (chars.:0)"=w280) -> ("all rows"=w269:string[][], "mark after read (chars.)"=w279:i32, "EOF?"=w274:bool)  [unwired: 7 in, 3 out]
          n122 = Build Array (concatenate)(w284, w283) -> (w282:string[])
          n123 = Index Array(array=w269, index (row)=0) -> (element=w267:string[])  [unwired: 1 in]
          n124 = Or(x=w273, y=w274) -> (x .or. y?=w272:bool)
          n125 = case shown="True" w273 {
            tunnel: [w286 w287] -> w271
            tunnel: w270 -> [w286 w291]
            tunnel: w282 -> [_ w289]
            tunnel: w267 -> [_ w288]
            frame False {
            }
            frame True {
              n126 = Build Array (concatenate)(w288, w289) -> (w290:string[])
              n127 = Build Array (concatenate)(w291, w290) -> (w287:string[][])
            }
          }
          n128 = local write "Processing"("Adding BIN Info to Data Array - 07") -> ()
        }
      }
      n129 = Build Array (concatenate)(w245, "Data_Filename") -> (w244:string[])
      n130 = Build Array (concatenate)(w236, w244) -> (w250:string[])
      n131 = Insert Into Array(array=w238, index (row)=0, new element=w250) -> (w241:string[][])  [unwired: 1 in]
      "BEST (Closest in Datafile) Array - String with BIN ASSIGNMENTS" <- w241
      n132 = case shown="True" "SAVE File" {
        tunnel: w241 -> [_ w296]
        tunnel: "SAVED Data BINS File Path Control" -> [_ w294]
        frame False {
        }
        frame True {
          n133 = call-poly <vilib>:"Write Delimited Spreadsheet.vi"("file path (dialog if empty)"=w294, "2D data"=w296) -> ("error out"=→"SAVE FILE error out":errorcluster)  [unwired: 12 in, 1 out]
        }
      }
    }
    frame #8 {
      # "Calculate STATISTICS for each column of independent data"
      # "Calculate Statistics on the BINNED Data Columns"
      n134 = Delete From Array "Delete From Array"(array=w300, index (row)=0) -> (array with subset deleted=w307:string[][])  [unwired: 2 in, 1 out]
      n135 = Fract/Exp String To Number(string=w307) -> (number=w303:dbl[][])  [unwired: 3 in, 1 out]
      n136 = Array Size(array=w303) -> (size(s)=w306:i32[])
      n137 = Transpose 2D Array(2D array=w300) -> (transposed array=w301:string[][])
      n138 = Transpose 2D Array(2D array=w303) -> (transposed array=w302:dbl[][])
      n139 = Index Array(array=w306, index=1) -> (element=w304:i32)
      n140 = for {
        N: w304 -> [_]
        tunnel: w302 -> [w320] mode=indexing
        tunnel: [w316] -> w298 mode=indexing
        tunnel: w301 -> [w315] mode=indexing
        n141 = Index Array(array=w315, index=0) -> (element=w313:string)
        n142 = call <vilib>:"Std Deviation and Variance.vi"("X"=w320) -> ("mean"=w322:dbl, "standard deviation"=w321:dbl)  [unwired: 1 in, 1 out]
        n143 = Array Max & Min(array=w320) -> (max value=w319:dbl, min value=w318:dbl)  [unwired: 2 out]
        n144 = Subtract(x=w319, y=w318) -> (x-y=w317:dbl)
        n145 = Bundle("String"=w313, "mean"=w322, "standard deviation"=w321, w319, w318, w317) -> (w316:T5)  [unwired: 1 in]
      }
      n146 = flat-sequence {
        tunnel: [w309] -> w299
        tunnel: w298 -> [w309]
        tunnel: [w311] -> w297
        tunnel: w299 -> [w311]
        frame #0 {
          n147 = local write "Processing"("Data Statistics Calc Done - 08") -> ()
        }
        frame #1 {
          n148 = Wait Until Next ms Multiple(millisecond multiple=u32 500) -> ()  [unwired: 1 out]
        }
      }
      "BINNED Data STATISTICS - Array" <- w297
    }
    frame #9 {
      # "Create the Sceenshots as JPGs."
      n149 = case shown="True" "Create PDF Report" {
        tunnel: w323 -> [_ w325]
        frame False {
        }
        frame True {
          n150 = stacked-sequence {
            seq-local: [w326 _ _ _] -> [_ _ _ w397]
            tunnel: w325 -> [w327 _ _ _]
            frame #0 {
              n151 = flat-sequence {
                frame #0 {
                  n152 = local write "Processing"("Creating PDF File of all LabView TABS - 9") -> ()
                }
                frame #1 {
                  n153 = Wait Until Next ms Multiple(millisecond multiple=u32 1000) -> ()  [unwired: 1 out]
                }
              }
              n154 = Path to Array of Strings(0:w327) -> (2:w341:string[])  [unwired: 1 out]
              n155 = Reverse 1D Array(array=w341) -> (reversed array=w336:string[])
              n156 = Index Array(array=w336, index=0) -> (element=w329:string)
              n157 = Delete From Array(array=w336, index=0) -> (array with subset deleted=w334:string[])  [unwired: 1 in, 1 out]
              n158 = call <vilib>:"Trim Whitespace.vi"("string"=w329) -> ("trimmed string"=w328:string)  [unwired: 1 in]
              n159 = Reverse 1D Array(array=w334) -> (reversed array=w332:string[])
              n160 = Match Pattern(string=w328, regular expression=".txt") -> (before substring=w339:string)  [unwired: 1 in, 3 out]
              n161 = Array of Strings to Path(0:w332) -> (2:w331:path)  [unwired: 1 in]
              n162 = Path To String(path=w331) -> (string=w330:string)
              n163 = Concatenate Strings("BINS_", w339, ".pdf") -> (w340:string)
              n164 = Concatenate Strings(w330, "\\", w340) -> (w333:string)
              "PDF Filename" <- w333
              n165 = String To Path(string=w333) -> (path=w326:path)
            }
            frame #1 {
              # "Manually change to equal number of tabs on front panel."
              n166 = for {
                N: 5 -> [_]
                i -> [w350]
                # "Start at Tab#"
                n167 = Current VI's Path() -> (path=w365:path)
                n168 = call <vilib>:"Trim Whitespace.vi"("string"="FDD") -> ("trimmed string"=w357:string)  [unwired: 1 in]
                n169 = Add(x=0, y=w350) -> (x+y=w349:i32)
                n170 = Open VI Reference(vi path=w365) -> (vi reference=w354:refnum<vi>, error out=w356:errorcluster)  [unwired: 1 in, 4 out]
                n171 = local write "Tab Control"(w349) -> ()
                n172 = flat-sequence {
                  tunnel: w356 -> [w379]
                  tunnel: [w379] -> w355
                  tunnel: w354 -> [w378]
                  tunnel: [w378] -> w353
                  frame #0 {
                    n173 = Wait Until Next ms Multiple(millisecond multiple=u32 1000) -> ()  [unwired: 1 out]
                  }
                }
                n174 = Number To Decimal String(number=w350) -> (decimal integer string=w363:string)  [unwired: 1 in]
                n175 = Concatenate Strings(w357, "_BIN_Plot0" ("string"), w363, ".jpg" ("string")) -> (w361:string)
                n176 = Build Array (concatenate)(string[] ["C", "Temp", "FDD_BIN_JPEGS"] ("array of strings"), w361) -> (w360:string[])
                n177 = flat-sequence {
                  tunnel: w352 -> [w375]
                  tunnel: [w375] -> w348
                  frame #0 {
                    n178 = Wait Until Next ms Multiple(millisecond multiple=u32 1000) -> ()  [unwired: 1 out]
                  }
                }
                n179 = Array of Strings to Path(0:w360) -> (2:w359:path)  [unwired: 1 in]
                n180 = invoke class="VI" method="FP.Get Image"(reference=w353, error in=w355, "visible area only"=FALSE ("Visible Area Only"), "image depth"=24 ("Image Depth")) -> (reference out=w367:refnum<vi>, error out=w369:errorcluster, "image data"=w370:T6)  [unwired: 2 in, 3 out]
                n181 = case shown="\"JPEG\", Default" enum16{"JPEG", "PNG", "BMP"}."JPEG" ("Image Type") {
                  tunnel: w370 -> [w383 w389 w393]
                  tunnel: w369 -> [w384 w388 w394]
                  tunnel: w359 -> [w382 w387 w392]
                  tunnel: [w380 w386 w391] -> w368
                  tunnel: w367 -> [w381 w385 w390]
                  tunnel: [w381 w385 w390] -> w366
                  frame "JPEG", Default {
                    n182 = call <vilib>:"Write JPEG File.vi"("error in (no error)"=w384, "image data"=w383, "path to JPEG file"=w382) -> ("error out"=w380:errorcluster)  [unwired: 8 out]
                  }
                  frame "PNG" {
                    n183 = call <vilib>:"Write PNG File.vi"("error in (no error)"=w388, "image data"=w389, "path to PNG file"=w387) -> ("error out"=w386:errorcluster)  [unwired: 8 out]
                  }
                  frame "BMP" {
                    n184 = call <vilib>:"Write BMP File.vi"("error in (no error)"=w394, "image data"=w393, "path to BMP file"=w392) -> ("error out"=w391:errorcluster)  [unwired: 8 out]
                  }
                }
                n185 = Close Reference(reference=w366, error in (no error)=w368) -> (error out=w352:errorcluster)
                "CREATE JPG error out" <- w348
              }
            }
            frame #2 {
              n186 = local write "Tab Control"(0) -> ()
            }
            frame #3 {
              w396 = TRUE  # overwrite (F)
              # "Create the PDF from the JPEG files."
              n187 = call <vilib>:"System Exec.vi"("run minimized? (F)"=TRUE, "command line"="C:\\Vance\\DAQ\\LabVIEW\\PDF Report BATCH File\\FDD_BIN_Report.bat") -> ("error out"=w398:errorcluster)  [unwired: 6 in, 3 out]
              n188 = Copy(8:w398, 9:w396, 10:w397, 11:path "C:/Temp/Blank_161207.pdf" ("source path")) -> ()  [unwired: 1 in, 3 out]
            }
          }
        }
      }
    }
  }
  n189 = local write "Running"(w12) -> ()
  "Running" <- TRUE ("Running")
  "Processing" <- "START" ("Processing")
